vi "TEST_AB_Application - Class Actor Framework.vi"() -> (0 "error description out":T1)   [LabVIEW 2023]
uses:
  utility.llb/array of error description.ctl
  utility.llb/error description.ctl
  utility.llb/error type.ctl
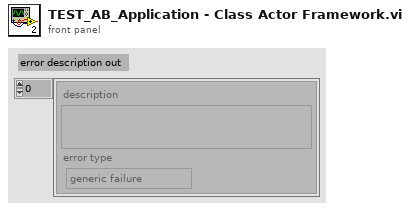
[diagram p1: front panel]
types:
  T1 = typedef "array of error description.ctl" = T2[]
  T2 = typedef "error description.ctl" = cluster{"description":string, "error type":T3}
  T3 = typedef "error type.ctl" = enum32{"generic failure", "boundary case", "precision", "expected error"}
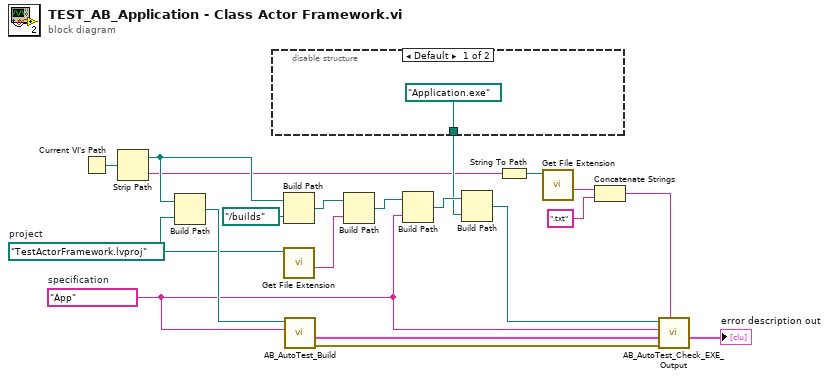
[diagram p0: block diagram]
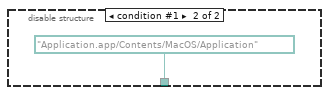
[diagram p2: hidden frame]
diagram:
  w5 = "App"  # specification
  w15 = path "TestActorFramework.lvproj"  # project
  n1 = Current VI's Path() -> (path=w20:path)
  n2 = Strip Path(path=w20) -> (stripped path=w18:path, name=w10:string)
  n3 = Build Path(base path=w18, name or relative path=w15) -> (appended path=w19:path)
  n4 = disable-structure shown="Default" {
    disable-tunnel: [path "Application.exe" ("Path") path "Application.app/Contents/MacOS/Application" ("Path")] -> w11
    frame condition #0 (active) {
    }
    frame condition #1 {
    }
  }
  n5 = Build Path(base path=w18, name or relative path=path "../builds") -> (appended path=w16:path)
  n6 = call <vilib>:"Get File Extension.vi"("file"=w15) -> ("filename without extension"=w14:string)  [unwired: 6 in, 4 out]
  n7 = call "AB_AutoTest_Build.vi"("BuildSpecName"=w5, "Project Name"=w19) -> ("error out"=w3:errorcluster, "error description out"=w4:T1)  [unwired: 7 in, 1 out]
  n8 = Build Path(base path=w16, name or relative path=w14) -> (appended path=w13:path)
  n9 = Build Path(base path=w13, name or relative path=w5) -> (appended path=w12:path)
  n10 = Build Path(base path=w12, name or relative path=w11) -> (appended path=w6:path)
  n11 = String To Path(string=w10) -> (path=w9:path)
  n12 = call <vilib>:"Get File Extension.vi"("file"=w9) -> ("filename without extension"=w8:string)  [unwired: 6 in, 4 out]
  n13 = Concatenate Strings(w8, ".txt" ("string")) -> (w2:string)
  n14 = call "AB_AutoTest_Check_EXE_Output.vi"("output filename"=w2, "error in (no error)"=w3, "error description in"=w4, "Build Spec Name"=w5, "EXE path"=w6) -> ("error description out"=→"error description out":T1)  [unwired: 5 in, 1 out]
